vi "manage loss communication.vi"(8 "error in (no error)":errorcluster, 11 "Channel in":refnum<class "SPARC4_Channel.lvclass">) -> (0 "error out":errorcluster, 3 "Channel out":refnum<class "SPARC4_Channel.lvclass">)   [LabVIEW 2018, in "SPARC4_Channel.lvclass"]
uses:
  SPARC4_Channel.lvclass
  Server/Server.lvclass
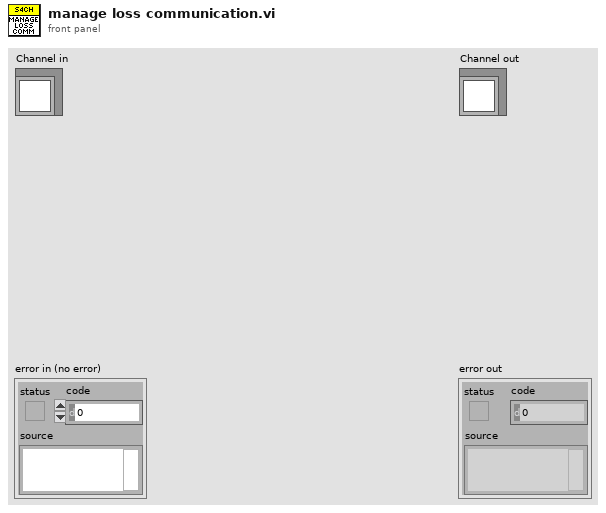
[diagram p1: front panel]
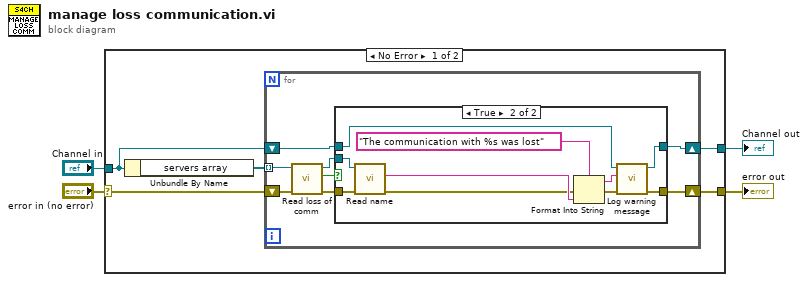
[diagram p0: block diagram]
diagram:
  n1 = case shown="No Error" "error in (no error)" {
    selector: "error in (no error)" -> [w8 w31]
    tunnel: [w7 w31] -> w3
    tunnel: [w6 w30] -> w1
    tunnel: "Channel in" -> [w9 w30]
    frame No Error {
      n2 = Unbundle By Name(w9) -> ("servers array"=w5:refnum<class "Server.lvclass">[])
      n3 = for {
        shift-right: [w16] -> w6
        shift-left: w9 -> [w17]
        shift-right: [w15] -> w7
        shift-left: w8 -> [w10]
        tunnel: w5 -> [w11] mode=indexing
        n4 = call-dynamic "Read loss of comm.vi"("error in (no error)"=w10, "Server in"=w11) -> ("error out"=w14:errorcluster, "loss of comm"=w13:bool, "Server out"=w12:refnum<class "Server.lvclass">)  [unwired: 7 in]
        n5 = case shown="True" w13 {
          tunnel: w17 -> [w19 w25]
          tunnel: [w19 w24] -> w16
          tunnel: [w18 w26] -> w15
          tunnel: w14 -> [w18 w23]
          tunnel: w12 -> [_ w22]
          frame False {
          }
          frame True {
            n6 = call-dynamic "Read name.vi"("error in (no error)"=w23, "Server in"=w22) -> ("error out"=w20:errorcluster, "name"=w21:string)  [unwired: 7 in, 1 out]
            n7 = Format Into String(format string="The communication with %s was lost", error in=w20, w21) -> (resulting string=w28:string, error out=w27:errorcluster)  [unwired: 1 in]
            n8 = call "Log warning message.vi"("error in (no error)"=w27, "String"=w28, "Channel in"=w25) -> ("error out"=w26:errorcluster, "Channel out"=w24:refnum<class "SPARC4_Channel.lvclass">)  [unwired: 7 in]
          }
        }
      }
    }
    frame Error {
    }
  }
  "error out" <- w3
  "Channel out" <- w1
